vi "Calling Python Script.vi"() -> ()   [LabVIEW 2017]
panel:
  in  "Path to Python.exe":path=path "C:/Python26/python.exe"
  out "Raw Python String Output":string
  out "Converted Output":i32
  in  "B":i32
  in  "A":i32
  out "error out":errorcluster
  out "Standard Error":string
  out "Return Code":i32
  # "1. Inputs - Set before running VI"
  # "2. Outputs"
  # "3. Errors - Both Standard and LabVIEW"
  # "A + B ="
  # "This VI sends inputs to a simple Python script, and returns its output.\n\nSee block diagram for code and comments"
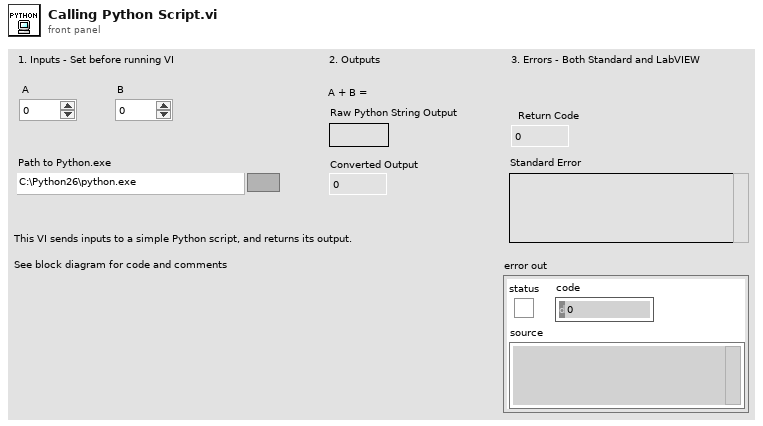
[diagram p1: front panel]
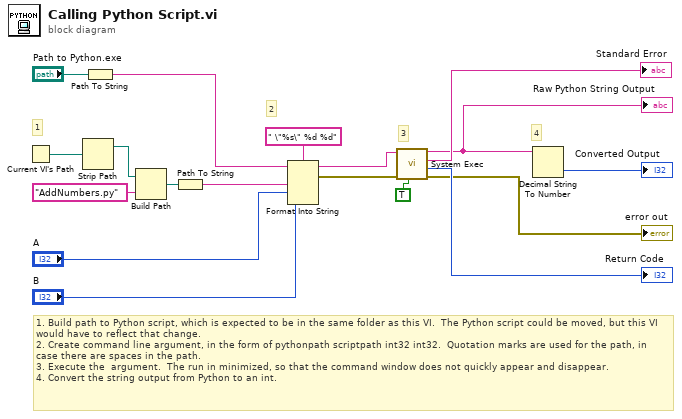
[diagram p0: block diagram]
diagram:
  # "1. Build path to Python script, which is expected to be in the same folder as this VI.  The Python script could be moved, but this VI would have to reflect that change.\n2. Create command line argument, in the form of pythonpath scriptpath int32 int32.  Quotation marks are used for the path, in case there are spaces in the path.\n3. Execute the  argument.  The run in minimized, so that the command window does not quickly appear and disappear.\n4. Convert the string output from Python to an int."
  # "4"
  # "3"
  # "2"
  # "1"
  n1 = Current VI's Path() -> (path=w8:path)
  n2 = Strip Path(path=w8) -> (stripped path=w5:path)  [unwired: 1 out]
  n3 = Path To String(path="Path to Python.exe") -> (string=w7:string)
  n4 = Build Path(base path=w5, name or relative path="AddNumbers.py" ("Path to Function")) -> (appended path=w13:path)
  n5 = Path To String(path=w13) -> (string=w14:string)
  n6 = Format Into String(format string=" \"%s\" %d %d", initial string=w7, w14, "A", "B") -> (resulting string=w11:string, error out=w9:errorcluster)  [unwired: 1 in]
  n7 = call <vilib>:"System Exec.vi"("run minimized? (F)"=TRUE, "error in (no error)"=w9, "command line"=w11) -> ("error out"=→"error out":errorcluster, "return code"=→"Return Code":i32, "standard error"=→"Standard Error":string, "standard output"=w4:string)  [unwired: 5 in]
  "Raw Python String Output" <- w4
  n8 = Decimal String To Number(string=w4) -> (number=→"Converted Output":i32)  [unwired: 2 in, 1 out]
